vi "tdmsGenToolExtended.vi"() -> ()   [LabVIEW 2026]
uses:
  <vilib>/platform/TimedLoop/XDataNode/XDataNode.xnode
  <vilib>/Platform/TimedLoop/XDataNode/nitl_modes.ctl
  <vilib>/Platform/TimedLoop/XDataNode/XDNodeRunTimeDep.lvlib
  <vilib>/Platform/TimedLoop/XDataNode/wakeup.ctl
  <vilib>/Platform/TimedLoop/XDataNode/timing_clust.ctl
  <vilib>/DAQmx/create/channels.llb/DAQmx Create Channel (AI-Voltage-Basic).vi
  <vilib>/DAQmx/configure/timing.llb/DAQmx Timing (Sample Clock).vi
  <vilib>/DAQmx/configure/task.llb/DAQmx Configure Logging (TDMS).vi
panel:
  in  "extended.":bool
  in  "file format version (2.0)":enum16{"1.0", "2.0"}(ring)=enum."2.0"
  in  "create index file? (T)":bool=TRUE
  in  "byte order (2:little-endian)":T1(ring)
  in  "physical channels":tag
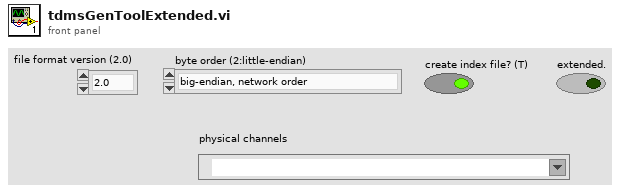
[diagram p1: front panel]
types:
  T1 = enum16{"big-endian, network order", "native, host order", "little-endian"}
  T2 = enum16{"open", "open or create", "create or replace", "create", "open (read-only)"}
  T3 = typedef "XDNodeRunTimeDep.lvlib/nitl_modes.ctl" = enum32{"No Change", "Process missed periods, maintain original phase", "Discard missed periods, maintain original phase", "Process missed periods, ignore original phase", "Discard missed periods, ignore original phase"}
  T4 = typedef "XDNodeRunTimeDep.lvlib/timing_clust.ctl" = cluster{"Expected End [f-1]":u64, "Actual End [f-1]":u64, "Finished Late? [f-1]":bool, "Expected End [i-1]":u64, "Actual End [i-1]":u64, "Finished Late? [i-1]":bool, "Expected Start [i]":u64, "Actual Start [i]":u64, "Expected Start [f]":u64, "Actual Start [f]":u64, "Source Name":string, "Structure Name":string, "Period":i64, "Deadline":i64, "Offset":i64, "Start":i64, "Priority":i32, "Timeout":i32, "Mode":T3, "Wakeup Reason":T5, "Error":errorcluster, "Source Type":string, "Secondary Source Type":string, "Global End Time":u64, "Global Start Time":u64, "Frame Duration":u64, "Iteration Duration":u64, "Assigned CPU":i32, "I/O Scan Engine Mode":u32}
  T5 = typedef "XDNodeRunTimeDep.lvlib/wakeup.ctl" = enum32{"Normal", "Aborted", "Asynchronous wakeup", "Timing source error", "Timed loop error", "Timeout"}
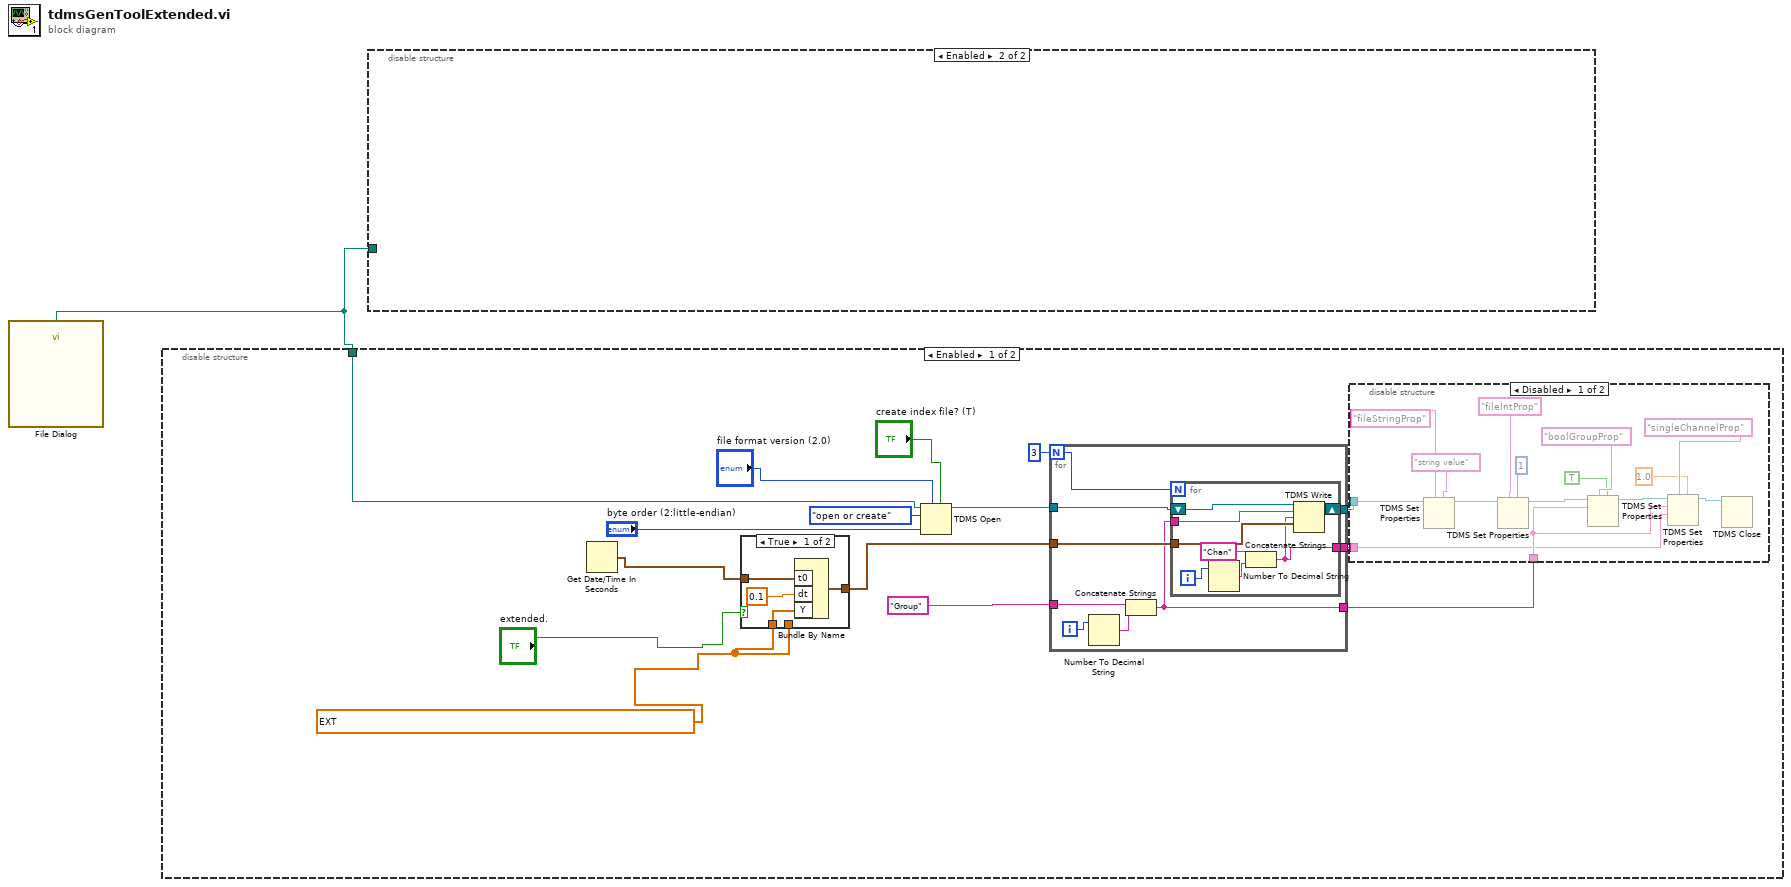
[diagram p0: block diagram]
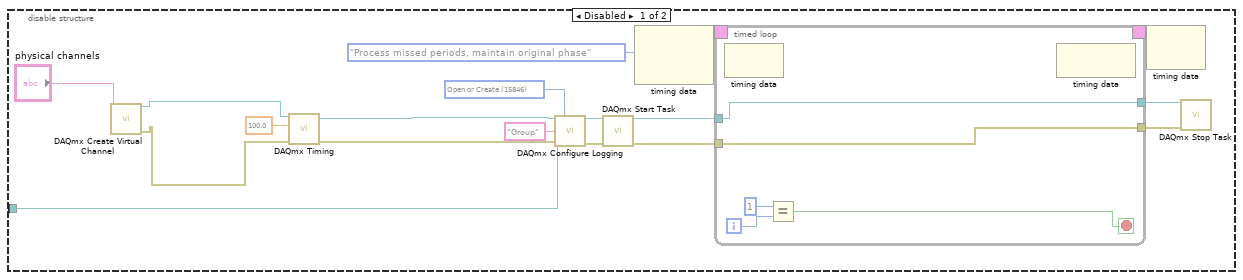
[diagram p2: hidden frame]
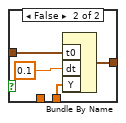
[diagram p4: hidden frame]
diagram:
  n1 = call "File Dialog"() -> ("selected path"=w1:path)  [unwired: 12 in, 3 out]
  n2 = disable-structure shown="Enabled" {
    disable-tunnel: w1 -> [w11 _]
    frame Enabled {
      w2 = ext[] [0.0, 1.0, 2.0, 3.0, 4.0, 5.0, 6.0, 7.0, 8.0, 9.0, 10.0] ("Y")
      n3 = Get Date/Time In Seconds() -> (seconds since 1Jan1904=w5:timestamp)
      n4 = case shown="True" "extended." {
        tunnel: w5 -> [w35 w39]
        tunnel: [w33 w37] -> w14
        tunnel: w2 -> [w32 _]
        tunnel: w2 -> [_ w36]
        frame True {
          n5 = Bundle By Name("t0"=w35, "dt"=0.1, "Y"=w32) -> (w33:waveform(ext))  [unwired: 1 in]
        }
        frame False {
          n6 = Bundle By Name("t0"=w39, "dt"=0.1, "Y"=w36) -> (w37:waveform(ext))  [unwired: 1 in]
        }
      }
      n7 = TDMS Open(5:"create index file? (T)", 7:"file format version (2.0)", 9:"byte order (2:little-endian)", 10:T2."open or create" ("operation (0:open)"), 11:w11) -> (3:w16:refnum<k34>)  [unwired: 2 in, 1 out]
      n8 = for {
        N: 3 -> [w42]
        tunnel: w16 -> [w48]
        tunnel: [w47] -> w6
        tunnel: "Group" ("String") -> [w45]
        tunnel: w14 -> [w43]
        tunnel: [w41] -> w4
        tunnel: [w40] -> w3
        i -> [w44]
        n9 = Number To Decimal String(number=w44) -> (decimal integer string=w46:string)  [unwired: 1 in]
        n10 = Concatenate Strings(w45, w46) -> (w41:string)
        n11 = for {
          N: w42 -> [_]
          tunnel: w41 -> [w54]
          shift-right: [w55] -> w47
          shift-left: w48 -> [w56]
          tunnel: w43 -> [w53]
          tunnel: [w49] -> w40
          i -> [w52]
          n12 = Number To Decimal String(number=w52) -> (decimal integer string=w51:string)  [unwired: 1 in]
          n13 = Concatenate Strings("Chan" ("string"), w51) -> (w49:string)
          n14 = TDMS Write(0:w56, 5:w54, 7:w49, 9:w53) -> (4:w55:refnum<k34>)  [unwired: 2 in, 3 out]
        }
      }
      n15 = disable-structure shown="Disabled" {
        disable-tunnel: w6 -> [w31 _]
        disable-tunnel: w4 -> [w18 _]
        disable-tunnel: w3 -> [w17 _]
        frame Disabled {
          n16 = TDMS Set Properties(5:"string value", 7:"fileStringProp", 11:w31) -> (3:w30:refnum<k34>)  [unwired: 3 in, 3 out]
          n17 = TDMS Set Properties(5:1 ("x"), 7:"fileIntProp", 11:w30) -> (3:w25:refnum<k34>)  [unwired: 3 in, 3 out]
          n18 = TDMS Set Properties(5:TRUE, 7:"boolGroupProp", 10:w18, 11:w25) -> (3:w22:refnum<k34>)  [unwired: 2 in, 3 out]
          n19 = TDMS Set Properties(5:sgl 1.0, 7:"singleChannelProp", 9:w17, 10:w18, 11:w22) -> (3:w21:refnum<k34>)  [unwired: 1 in, 3 out]
          n20 = TDMS Close(11:w21) -> ()  [unwired: 1 in, 2 out]
        }
        frame Enabled {
        }
      }
    }
    frame Disabled {
    }
  }
  n21 = disable-structure shown="Enabled" {
    disable-tunnel: w1 -> [w60 _]
    frame Disabled {
      w71 = 15846 items=["Open"=10437, "Open or Create"=15846, "Create or Replace"=15847, "Create"=15848] ("operation")
      n22 = call-poly <vilib>:"DAQmx Create Virtual Channel.vi"("physical channels"="physical channels") -> ("task out"=w59:refnum<k21>, "error out"=w58:errorcluster)  [unwired: 13 in]
      n23 = call-poly <vilib>:"DAQmx Timing.vi"("task/channels in"=w59, "rate"=100.0, "error in"=w58) -> ("task out"=w69:refnum<k21>, "error out"=w68:errorcluster)  [unwired: 11 in]
      n24 = call-poly <vilib>:"DAQmx Configure Logging.vi"("task/channels in"=w69, "operation"=w71, "file path"=w60, "group name"="Group", "error in"=w68) -> ("task out"=w67:refnum<k21>, "error out"=w66:errorcluster)  [unwired: 9 in]
      n25 = call <vilib>:"DAQmx Start Task.vi"("task/channels in"=w67, "error in"=w66) -> ("task out"=w65:refnum<k21>, "error out"=w64:errorcluster)  [unwired: 12 in]
      n26 = node-c288(nitl_modes."Process missed periods, maintain original phase" ("Mode")) -> (w74:T4)  [unwired: 1 in]
      n27 = timed-loop {
        tunnel: w65 -> [w76]
        tunnel: w64 -> [w75]
        timing: w74 -> [_]
        timing-out: [_] -> w73
        tunnel: [w76] -> w63
        tunnel: [w75] -> w62
        i -> [w79]
        stop <- w77 stop-if-true
        n28 = node-c288() -> ()  [unwired: 1 in, 1 out]
        n29 = Equal?(x=1, y=w79) -> (x = y?=w77:bool)
        n30 = node-c288() -> ()  [unwired: 1 in, 1 out]
      }
      n31 = node-c288(w73) -> ()  [unwired: 1 out]
      n32 = call <vilib>:"DAQmx Stop Task.vi"("task/channels in"=w63, "error in"=w62) -> ()  [unwired: 12 in, 2 out]
    }
    frame Enabled {
    }
  }
